vi "Igor_wave_colors.vi"(1 "Array":string[](array[string])) -> (0 "concatenated string":string)   [LabVIEW 2021]
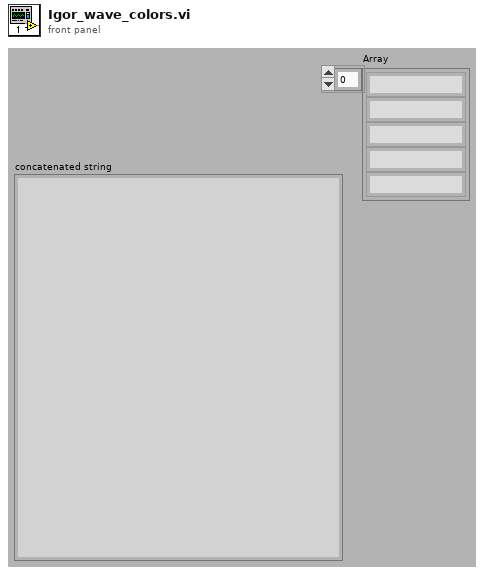
[diagram p1: front panel]
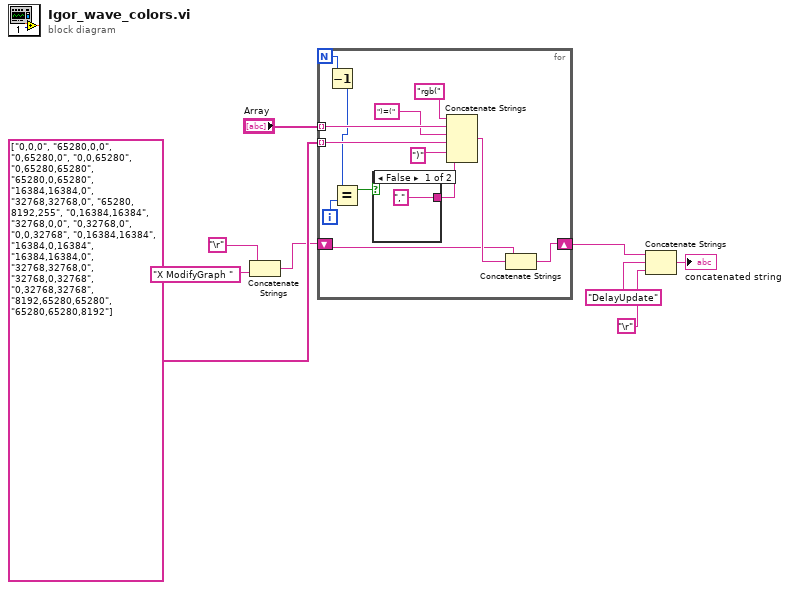
[diagram p0: block diagram]
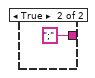
[diagram p2: hidden frame]
diagram:
  n1 = Concatenate Strings("\r", "X ModifyGraph " ("string")) -> (w1:string)
  n2 = for {
    N -> [w14]
    tunnel: "Array" -> [w22] mode=indexing
    tunnel: string[] ["0,0,0", "65280,0,0", "0,65280,0", "0,0,65280", "0,65280,65280", "65280,0,65280", "16384,16384,0", "32768,32768,0", "65280, 8192,255", "0,16384,16384", "32768,0,0", "0,32768,0", "0,0,32768", "0,16384,16384", "16384,0,16384", "16384,16384,0", "32768,32768,0", "32768,0,32768", "0,32768,32768", "8192,65280,65280", "65280,65280,8192"] -> [w20] mode=indexing
    shift-right: [w11] -> w7
    shift-left: w1 -> [w10]
    i -> [w15]
    n3 = Decrement(x=w14) -> (x-1=w13:i32)
    n4 = Equal?(x=w13, y=w15) -> (x = y?=w16:bool)
    n5 = case shown="False" w16 {
      tunnel: ["," ("string") ";" ("string")] -> w17
      frame False {
      }
      frame True {
      }
    }
    n6 = Concatenate Strings("rgb(" ("string"), w22, ")=(" ("string"), w20, ")" ("string"), w17) -> (w12:string)
    n7 = Concatenate Strings(w10, w12) -> (w11:string)
  }
  n8 = Concatenate Strings(w7, "DelayUpdate" ("string"), "\r") -> (→"concatenated string":string)
